vi "WayPointFollowing.vi"() -> ()   [LabVIEW 2010]
uses:
  <vilib>/gmath/NI_Gmath.lvlib
  <vilib>/gmath/statdist.llb/Normal PDF.vi
  <vilib>/Analysis/NI_AALBase.lvlib
  <vilib>/Analysis/1siggen.llb/Ramp Pattern by Samples.vi
  5.0-Global.vi
panel:
  out "Where-to-Where In Indicator":T1(array[cluster])
  out "Where-to-Where Out Indicator":T1(array[cluster])
  out "ActCommand":dbl[](array[numeric])
  in  "InhibitIn":bool
  in  "SupressIn":dbl=1.0
  out "SupressOut":dbl
  out "loop index":i32
  out "InhibitOut":bool
  out "Vel":dbl
  out "SteerAngle":dbl
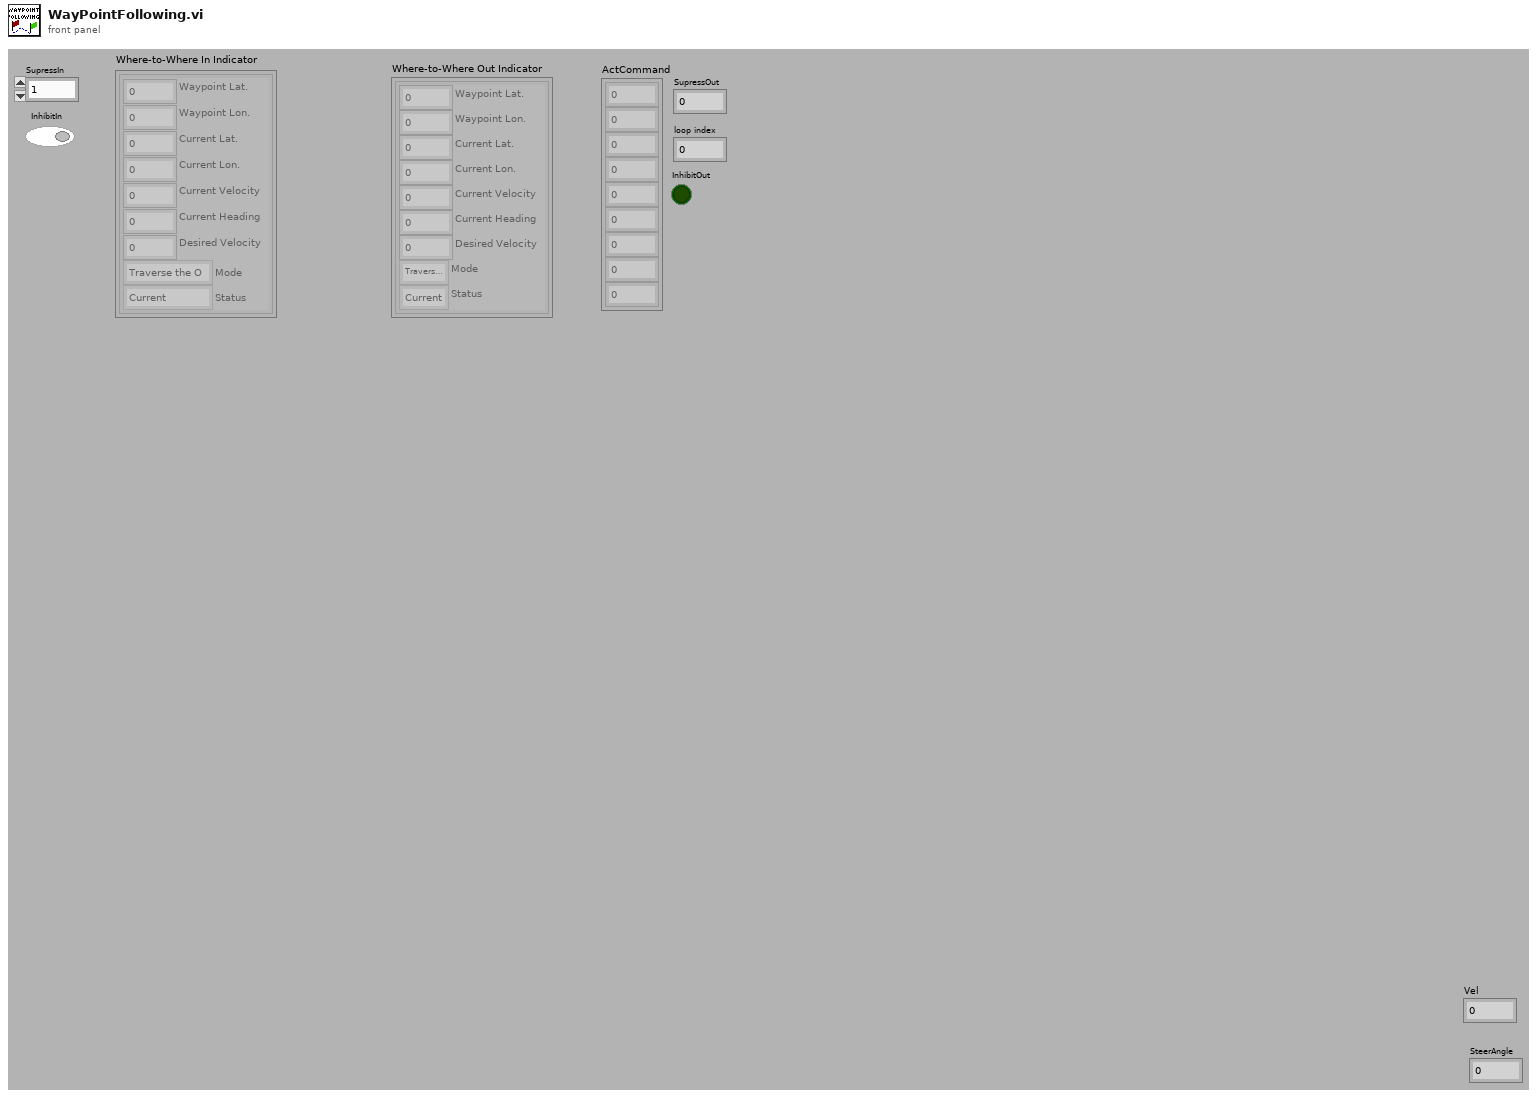
[diagram p1: front panel]
types:
  T1 = cluster{"Waypoint Lat.":dbl, "Waypoint Lon.":dbl, "Current Lat.":dbl, "Current Lon. ":dbl, "Current Velocity":dbl, "Current Heading":dbl, "Desired Velocity":dbl, "Mode":enum16{"Traverse the O"}, "Status":enum16{"Current", "Future", "Past"}}[]
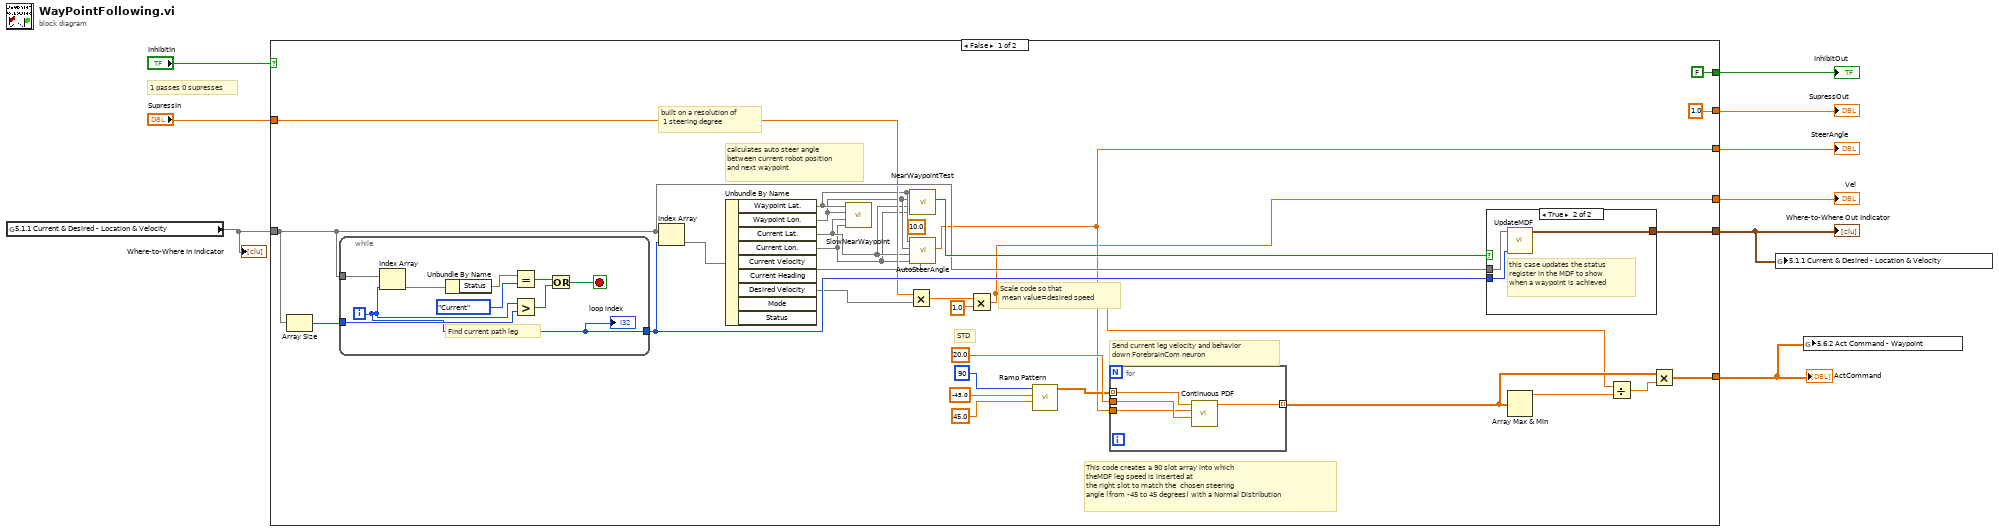
[diagram p0: block diagram]
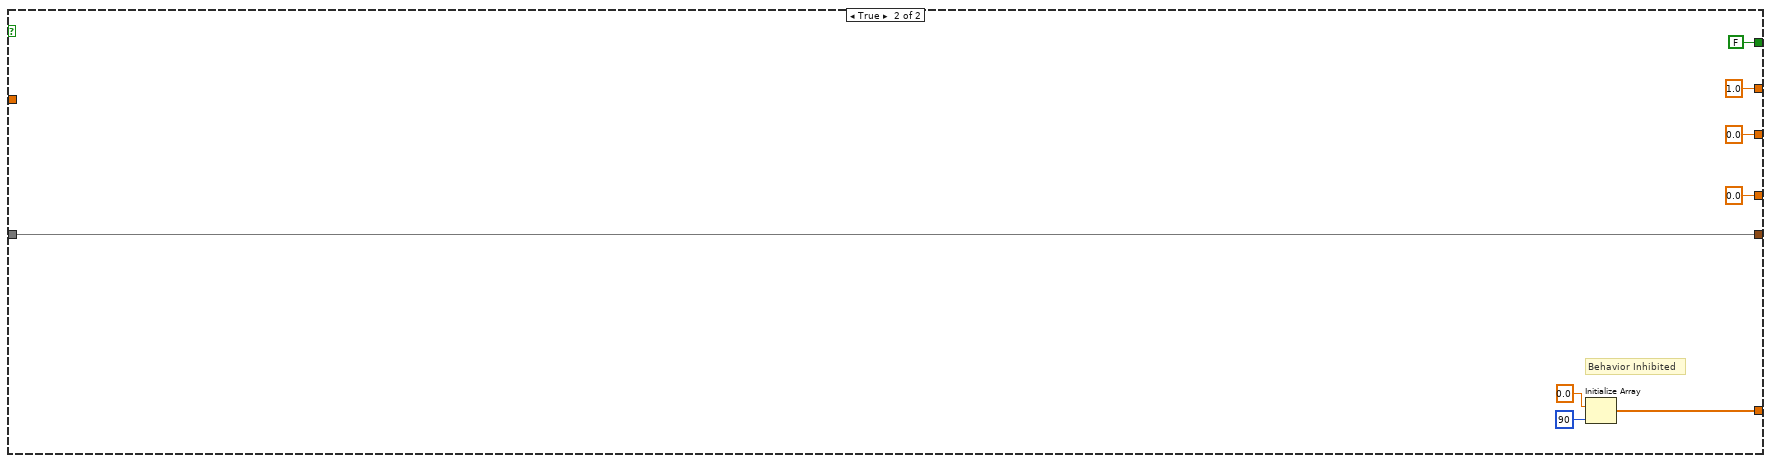
[diagram p3: hidden frame]
diagram:
  # "1 passes 0 supresses"
  n1 = global read "5.0-Global.vi" "5.1.1 Current & Desired - Location & Velocity"() -> (w3)
  "Where-to-Where In Indicator" <- w3
  n2 = case shown="False" "InhibitIn" {
    tunnel: "SupressIn" -> [w20 _]
    tunnel: [w26 w60] -> w1
    tunnel: [1.0 ("SupressOut") 1.0 ("SupressOut")] -> w6
    tunnel: [FALSE ("InhibitOut") FALSE ("InhibitOut")] -> w7
    tunnel: w3 -> [w24 w57]
    tunnel: [w23 w57] -> w2
    tunnel: [w10 0.0 ("Vel")] -> w8
    tunnel: [w21 0.0 ("SteerAngle")] -> w9
    frame False {
      (unwired) 10.0 ("Capture Radius")
      # "calculates auto steer angle\nbetween current robot position\nand next waypoint"
      # "built on a resolution of\n 1 steering degree"
      # "Scale code so that\n mean value=desired speed"
      # "STD"
      # "This code creates a 90 slot array into which\ntheMDF leg speed is inserted at\nthe right slot to match the  chosen steering\nangle (from -45 to 45 degrees) with a Normal Distribution"
      # "Send current leg velocity and behavior\ndown ForebrainCom neuron"
      n3 = Array Size(array=w24) -> (size(s)=w35:i32)
      n4 = while {
        tunnel: w35 -> [w54]
        tunnel: w24 -> [w51]
        tunnel: [w47] -> w22
        i -> [w47]
        stop <- w53 stop-if-true
        # "Find current path leg"
        n5 = Index Array "Index Array"(array=w51, index=w47) -> (element=w48)
        n6 = Unbundle By Name(w48) -> ("Status"=w49)
        n7 = Equal?(x=w49, y=enum16{"Current", "Future", "Past"}."Current") -> (x = y?=w50:bool)
        n8 = Greater?(x=w47, y=w54) -> (0:w52:bool)
        n9 = Or(x=w50, y=w52) -> (x .or. y?=w53:bool)
        "loop index" <- w47
      }
      n10 = Index Array "Index Array"(array=w24, index=w22) -> (element=w17)
      n11 = Unbundle By Name(w17) -> ("Waypoint Lat."=w15, "Waypoint Lon."=w14, "Current Lat."=w13, "Current Lon."=w12, "Current Heading"=w11, "Desired Velocity"=w16)  [unwired: 3 out]
      n12 = call "SlowNearWaypoint.vi"("Current Lon."=w12, "Current Lat."=w13, "Waypoint Lon."=w14, "Waypoint Lat."=w15) -> ()  [unwired: 2 in, 1 out]
      n13 = Multiply(x=w20, y=w16) -> (x*y=w19:dbl)
      n14 = call "NearWaypointTest.vi"("Current Lon."=w12, "Current Lat."=w13, "Waypoint Lon."=w14, "Waypoint Lat."=w15) -> ("AtWaypoint"=w25:bool)  [unwired: 7 in]
      n15 = call "AutoSteerAngle.vi"("CurrentDirection"=w11, "Ycurrent"=w12, "Xcurrent"=w13, "Ywaypoint"=w14, "Xwaypoint"=w15) -> ("NewSteerAngle"=w21:dbl)  [unwired: 6 in]
      n16 = Multiply(x=w19, y=1.0) -> (x*y=w10:dbl)
      n17 = call-poly <vilib>:"Ramp Pattern.vi"("start"=45.0, "end"=-45.0 ("end (Normal)"), "samples"=90) -> ("Ramp Pattern"=w29:dbl[])  [unwired: 7 in, 1 out]
      n18 = for {
        tunnel: w29 -> [w45] mode=indexing
        tunnel: 20.0 ("std (Normal)") -> [w44]
        tunnel: [w43] -> w33 mode=indexing
        tunnel: w21 -> [w42]
        n19 = call-poly <vilib>:"Continuous PDF.vi"("std"=w44, "mean"=w42, "x"=w45) -> ("pdf(x)"=w43:dbl)  [unwired: 7 in, 1 out]
      }
      n20 = case shown="True" w25 {
        tunnel: w24 -> [w38 w40]
        tunnel: [w38 w39] -> w23
        tunnel: w22 -> [_ w41]
        frame False {
          # "robot not near waypoint\npass MDF through unaltered"
        }
        frame True {
          # "this case updates the status\nregister in the MDF to show \nwhen a waypoint is achieved"
          n21 = call "UpdateMDF.vi"("Index"=w41, "Where-to-Where In"=w40) -> ("Where-to-Where updated"=w39:T1)  [unwired: 9 in]
        }
      }
      n22 = Array Max & Min(array=w33) -> (max value=w31:dbl)  [unwired: 3 out]
      n23 = Divide(x=w10, y=w31) -> (x/y=w32:dbl)
      n24 = Multiply(x=w33, y=w32) -> (x*y=w26:dbl[])
    }
    frame True {
      # "Behavior Inhibited"
      n25 = Initialize Array "Initialize Array"(0.0 ("element"), 90 ("dimension size")) -> (w60:dbl[])
    }
  }
  "ActCommand" <- w1
  "SupressOut" <- w6
  "InhibitOut" <- w7
  "Vel" <- w8
  "SteerAngle" <- w9
  "Where-to-Where Out Indicator" <- w2
  n26 = global write "5.0-Global.vi" "5.1.1 Current & Desired - Location & Velocity"(w2) -> ()
  n27 = global write "5.0-Global.vi" "5.6.2 Act Command - Waypoint"(w1) -> ()
